vi "Init.vi"(6 "timeout (10000)":i32, 8 "error in (no error)":errorcluster, 10 "Auth token":string) -> (0 "error out":errorcluster, 3 "ByteQXAPIBase out":refnum<class "ByteQXAPIBase.lvclass">)   [LabVIEW 2019, in "ByteQXWebAPI.lvlib" / "ByteQXAPIBase.lvclass"]
uses:
  ByteQXAPIBase.lvclass
  <vilib>/Bytelabs/ByteREST/ByteRESTClass/ByteRESTBase/RESTBase.lvclass
  <vilib>/Bytelabs/ByteREST/CfgLoaders/LoaderBase/ServerParams.ctl
  <vilib>/Bytelabs/ByteREST/ByteRESTClass/ByteRESTBase/Auth/Authentication_type.ctl
  <vilib>/Bytelabs/ByteREST/CfgLoaders/LoaderConstant/RESTLoaderConstant.lvclass/RESTLoaderConstant.ctl
  ByteQXAPIBase.lvclass/ByteQXAPIBase.ctl
  <vilib>/Bytelabs/ByteREST/CfgLoaders/LoaderConstant/RESTLoaderConstant.lvclass
  C:/Program Files (x86)/National Instruments/LabVIEW 2019/vi.lib/Bytelabs/ByteREST/CfgLoaders/LoaderBase/RESTLoaderBase.lvclass
  <vilib>/Bytelabs/ByteREST/CfgLoaders/LoaderBase/RESTLoaderBase.lvclass
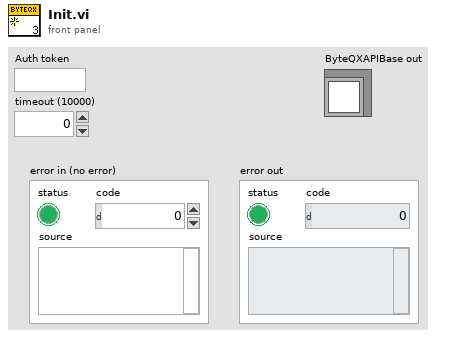
[diagram p1: front panel]
types:
  T1 = typedef "ByteREST.lvlib/RESTLoaderBase.lvclass/ServerParams.ctl" = cluster{"API Root":string, "verify server":bool, "Version (no version)":string, "Port (protocol specific)":u16, "Base URL":string, "Auth type":T2, "Auth string":string, "timeout (10000)":i32, "Token preamble (Token)":string, "Token empty preamble (False)":bool, "Token header key (Authorization)":string}
  T2 = typedef "ByteREST.lvlib/RESTBase.lvclass/Authentication_type.ctl" = enum16{"Token"}
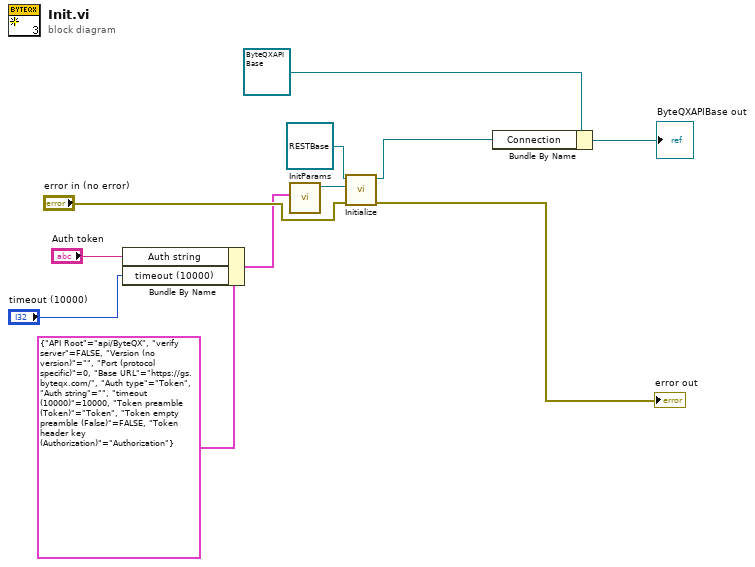
[diagram p0: block diagram]
diagram:
  n1 = Bundle By Name(cluster=T1 {"API Root"="api/ByteQX", "verify server"=FALSE, "Version (no version)"="", "Port (protocol specific)"=0, "Base URL"="https://gs.byteqx.com/", "Auth type"=enum."Token", "Auth string"="", "timeout (10000)"=10000, "Token preamble (Token)"="Token", "Token empty preamble (False)"=FALSE, "Token header key (Authorization)"="Authorization"} ("Cluster"), "Auth string"="Auth token", "timeout (10000)"="timeout (10000)") -> (w6:T1)
  n2 = call <vilib>:"InitParams.vi"("Cluster"=w6) -> ("RESTLoaderConstant out"=w8:refnum<class "RESTLoaderConstant.lvclass">)  [unwired: 10 in]
  n3 = call-dynamic "Initialize.vi"("error in (no error)"="error in (no error)", "RESTLoader"=w8, "REST in"=refnum<class "RESTBase.lvclass"> refnum) -> ("error out"=→"error out":errorcluster, "REST out"=w1:refnum<class "RESTBase.lvclass">)  [unwired: 7 in]
  n4 = Bundle By Name(cluster=refnum<class "ByteQXAPIBase.lvclass"> refnum ("ByteQXAPIBase in"), "Connection"=w1) -> (→"ByteQXAPIBase out":refnum<class "ByteQXAPIBase.lvclass">)
